vi "generate macro.autosave.path.vi"(8 "error in (no error)":errorcluster) -> (0 "error out":errorcluster, 3 "macro.autosave.path":path)   [LabVIEW 2012]
doc: "SciScan 1.2 160622"
uses:
  GFG/GFGpathGet.vi
  GFG/GFG library.lvlib
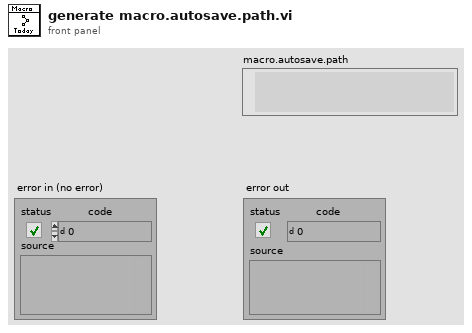
[diagram p1: front panel]
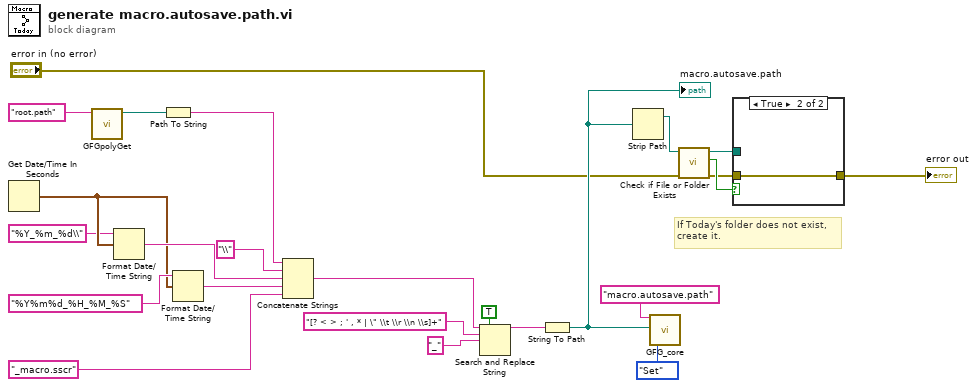
[diagram p0: block diagram]
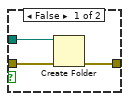
[diagram p2: hidden frame]
diagram:
  # "If Today's folder does not exist,\ncreate it."
  n1 = Get Date/Time In Seconds() -> (seconds since 1Jan1904=w13:timestamp)
  n2 = call-poly "GFGpolyGet.vi"("Variable Name in"="root.path") -> ("Path"=w17:path)  [unwired: 8 in, 2 out]
  n3 = Format Date/Time String(time format string (%c)="%Y_%m_%d\\", seconds (now)=w13) -> (date/time string=w14:string)  [unwired: 1 in]
  n4 = Path To String(path=w17) -> (string=w10:string)
  n5 = Format Date/Time String(time format string (%c)="%Y%m%d_%H_%M_%S", seconds (now)=w13) -> (date/time string=w15:string)  [unwired: 1 in]
  n6 = Concatenate Strings(w10, "\\" ("string"), w14, w15, "_macro.sscr" ("string")) -> (w9:string)
  n7 = Search and Replace String(replace all?=TRUE ("replace all? (F)"), input string=w9, search string="[? < > ; ' , * | \" \\t \\r \\n \\s]+", replace string="_" ("replace string (\"\")")) -> (result string=w23:string)  [unwired: 4 in, 3 out]
  n8 = String To Path(string=w23) -> (path=w7:path)
  "macro.autosave.path" <- w7
  n9 = Strip Path(path=w7) -> (stripped path=w6:path)  [unwired: 1 out]
  n10 = call "GFG_core.vi"("Variable Name in"="macro.autosave.path" ("Tag in"), "Variant in"=w7, "Action"=enum16{"Init", "Set", "Get"}."Set") -> ()  [unwired: 10 in, 7 out]
  n11 = call <vilib>:"Check if File or Folder Exists.vi"("error in (no error)"="error in (no error)", "path"=w6) -> ("error out"=w3:errorcluster, "file or folder exists?"=w5:bool, "dup path"=w4:path)  [unwired: 7 in]
  n12 = case shown="True" w5 {
    tunnel: w4 -> [w27 _]
    tunnel: w3 -> [w26 w28]
    tunnel: [w25 w28] -> w2
    frame False {
      n13 = Create Folder(path (use dialog)=w27, error in=w26) -> (error out=w25:errorcluster)  [unwired: 1 in, 2 out]
    }
    frame True {
    }
  }
  "error out" <- w2
